vi "Generate Error.vi"(8 "Error In":errorcluster, 10 "Adept Error Code":i32, 11 "DPCUTIL Error":T1) -> (0 "Error Out":errorcluster)   [LabVIEW 2011, in "LVH-Adept.lvlib" / "DPCUTIL.lvlib"]
uses:
  DPCUTIL.lvlib
  Type Defs/Error.ctl
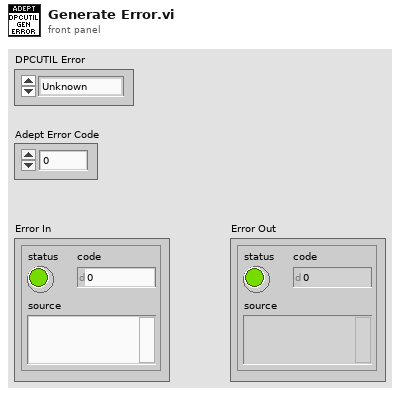
[diagram p1: front panel]
types:
  T1 = typedef "LVH-Adept.lvlib/DPCUTIL.lvlib/Error.ctl" = enum16{"Unknown", "Open Data", "Wait For Transaction", "Put Reg", "Get Reg", "Close Data"}
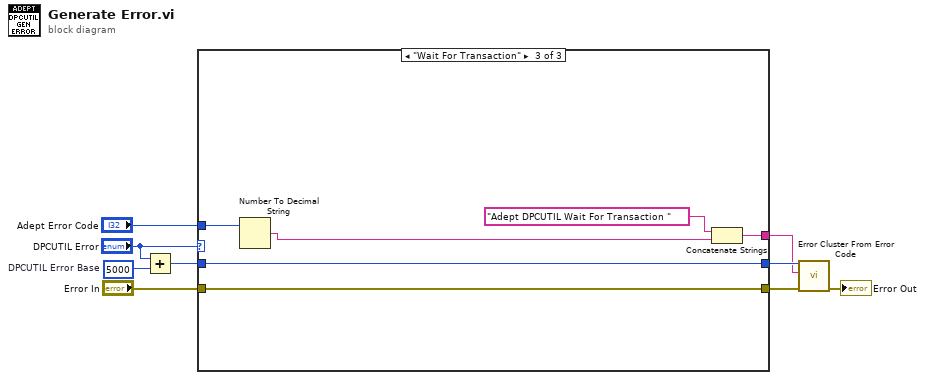
[diagram p0: block diagram]
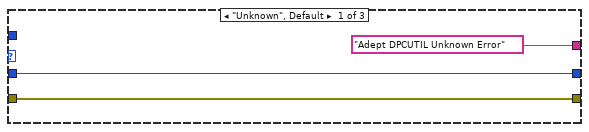
[diagram p2: hidden frame]
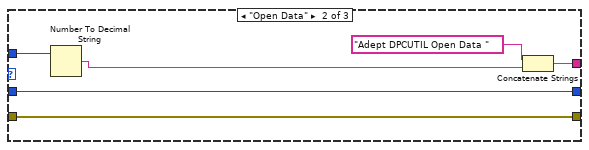
[diagram p3: hidden frame]
diagram:
  w8 = 5000  # DPCUTIL Error Base
  n1 = Add(x="DPCUTIL Error", y=w8) -> (x+y=w4:i32)
  n2 = case shown="\"Wait For Transaction\"" "DPCUTIL Error" {
    tunnel: [w12 w18 w24] -> w7
    tunnel: "Error In" -> [w12 w18 w24]
    tunnel: [w11 w17 w23] -> w5
    tunnel: w4 -> [w11 w17 w23]
    tunnel: ["Adept DPCUTIL Unknown Error" w13 w19] -> w2
    tunnel: "Adept Error Code" -> [_ w15 w21]
    frame "Unknown", Default {
    }
    frame "Open Data" {
      n3 = Number To Decimal String(number=w15) -> (decimal integer string=w14:string)  [unwired: 1 in]
      n4 = Concatenate Strings("Adept DPCUTIL Open Data ", w14) -> (w13:string)
    }
    frame "Wait For Transaction" {
      n5 = Number To Decimal String(number=w21) -> (decimal integer string=w20:string)  [unwired: 1 in]
      n6 = Concatenate Strings("Adept DPCUTIL Wait For Transaction ", w20) -> (w19:string)
    }
  }
  n7 = call <vilib>:"Error Cluster From Error Code.vi"("error in (no error)"=w7, "error message (\"\")"=w2, "error code (0)"=w5) -> ("error out"=→"Error Out":errorcluster)  [unwired: 6 in]
